vi "test_CCDSetRoi.vi"(0 "device selection":enum16{"monochromator", "CCD", "SCD"}(ring)=enum."CCD", 1 "Test should pass":bool=TRUE, 5 "set-up a connection":bool=TRUE, 9 "tear down connection":bool=TRUE, 11 "error in":errorcluster, 12 "activate logger?":bool, 13 "Handler Name":string="example logger handler") -> (2 "ready":bool, 3 "log-file path":path, 15 "error out":errorcluster)   [LabVIEW 2023]
uses:
  Classes/CCD/CCD.lvclass
  <vilib>/addons/_JKI Toolkits/Caraya/classes/Assert/Assert Not Error.vi
  <vilib>/addons/_JKI Toolkits/Caraya/classes/Test/Test.lvclass
  <vilib>/addons/_JKI Toolkits/Caraya/classes/Assert/Assert.lvclass
  C:/Projects/Horiba/horiba-labview-sdk/Source/Classes/GenericDevice/GenericDevice.lvclass
  C:/Projects/Horiba/horiba-labview-sdk/Source/Classes/CCD/CCD.lvclass
panel:
  in  "Delay between send and receive [ms]":i32=100
  out "config-JSON string":string
  # "Connector Pane"
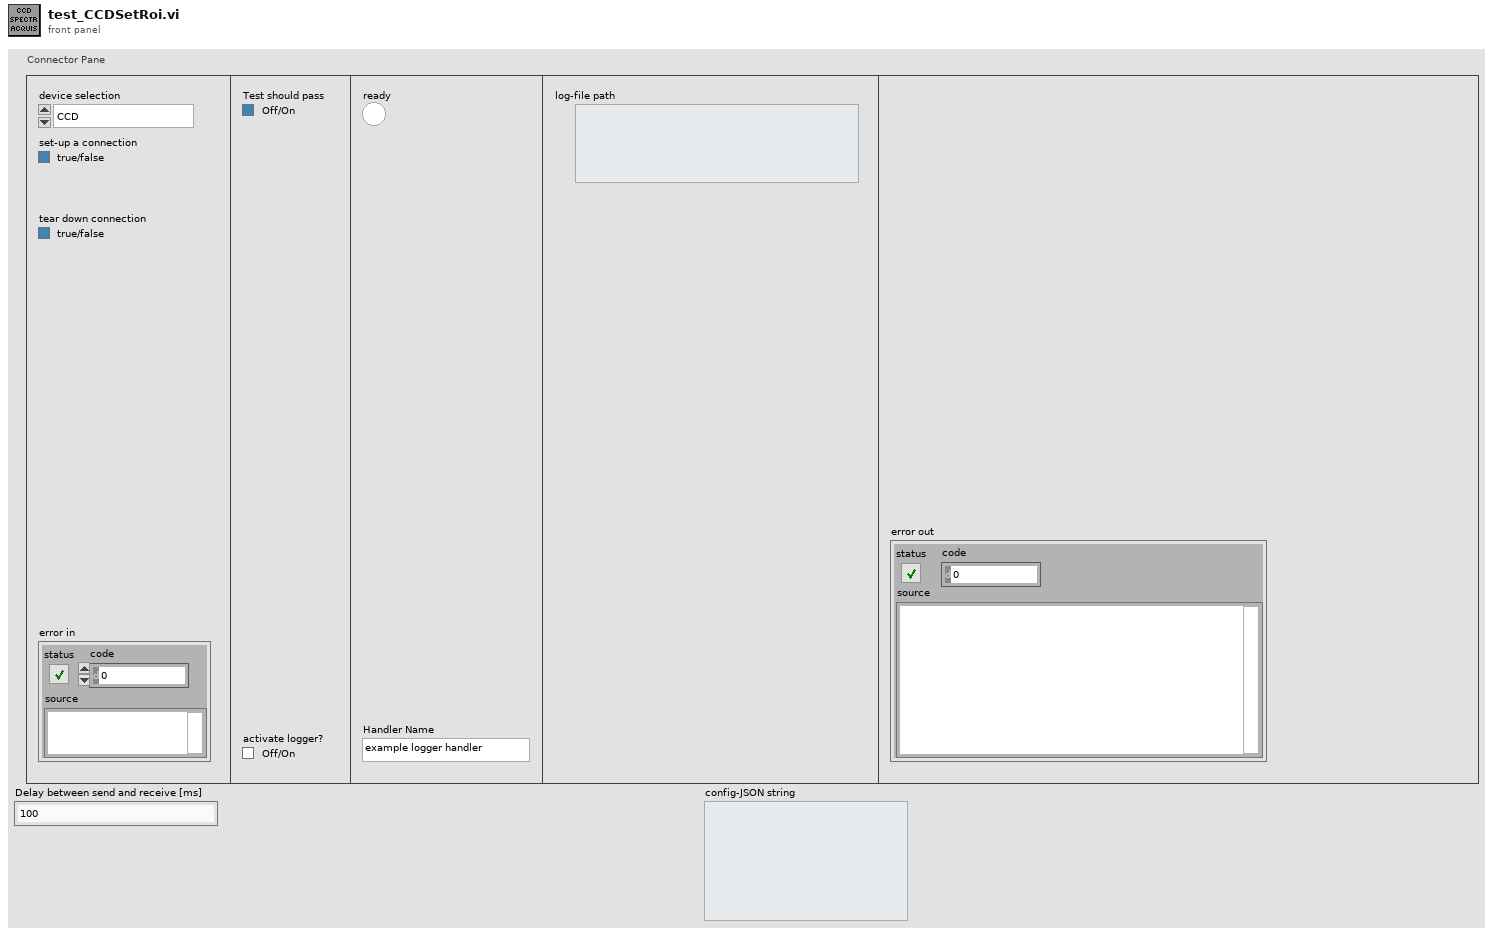
[diagram p1: front panel]
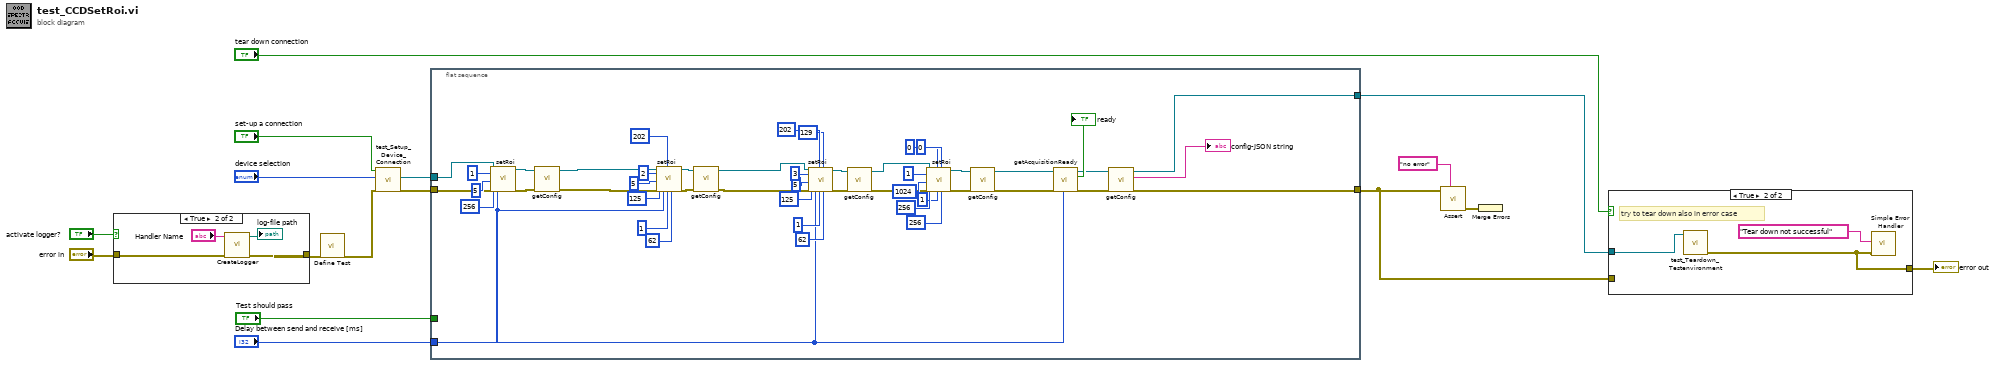
[diagram p0: block diagram]
diagram:
  n1 = case shown="True" "activate logger?" {
    tunnel: [w17 w20] -> w2
    tunnel: "error in" -> [w17 w21]
    frame False {
    }
    frame True {
      n2 = call "CreateLogger.vi"("error in (no error)"=w21, "Handler Name"="Handler Name") -> ("error out"=w20:errorcluster, "log-file path"=→"log-file path":path)  [unwired: 8 in]
    }
  }
  n3 = call <vilib>:"Define Test.vi"("error in (no error)"=w2) -> ("error out"=w7:errorcluster)  [unwired: 9 in, 1 out]
  n4 = call "test_Setup_Device_Connection.vi"("error in (no error)"=w7, "device selection"="device selection", "set-up a connection"="set-up a connection") -> ("error out"=w8:errorcluster, "CCD.lvclass"=w9:refnum<class "CCD.lvclass">)  [unwired: 5 in, 2 out]
  n5 = flat-sequence {
    tunnel: w8 -> [w52]
    tunnel: w9 -> [w36]
    tunnel: [w50] -> w12
    tunnel: "Test should pass" -> [w70]
    tunnel: [w48] -> w11
    tunnel: "Delay between send and receive [ms]" -> [w22]
    frame #0 {
      n6 = call "setRoi.vi"("CCD in"=w36, "ROI-index"=1, "xSize"=5, "ySize"=256, "error in (no error)"=w52, "Delay between send and receive [ms]"=w22) -> ("CCD out"=w40:refnum<class "CCD.lvclass">, "error out"=w39:errorcluster)  [unwired: 10 in, 2 out]
      n7 = call "getConfig.vi"("error in (no error)"=w39, "CCD in"=w40) -> ("error out"=w37:errorcluster, "CCD out"=w38:refnum<class "CCD.lvclass">)  [unwired: 7 in, 1 out]
      n8 = call "setRoi.vi"("CCD in"=w38, "ROI-index"=2, "xSize"=5, "ySize"=125, "error in (no error)"=w37, "Delay between send and receive [ms]"=w22, "xOrigin"=202, "xBin"=1, "yBin"=62) -> ("CCD out"=w43:refnum<class "CCD.lvclass">, "error out"=w44:errorcluster)  [unwired: 7 in, 2 out]
      n9 = call "getConfig.vi"("error in (no error)"=w44, "CCD in"=w43) -> ("error out"=w41:errorcluster, "CCD out"=w42:refnum<class "CCD.lvclass">)  [unwired: 7 in, 1 out]
      n10 = call "setRoi.vi"("CCD in"=w42, "ROI-index"=3, "xSize"=5, "ySize"=125, "error in (no error)"=w41, "Delay between send and receive [ms]"=w22, "xOrigin"=202, "xBin"=1, "yOrigin"=129, "yBin"=62) -> ("CCD out"=w45:refnum<class "CCD.lvclass">, "error out"=w46:errorcluster)  [unwired: 6 in, 2 out]
      n11 = call "getConfig.vi"("error in (no error)"=w46, "CCD in"=w45) -> ("error out"=w28:errorcluster, "CCD out"=w30:refnum<class "CCD.lvclass">)  [unwired: 7 in, 1 out]
      n12 = call "setRoi.vi"("CCD in"=w30, "ROI-index"=1, "xSize"=1024, "ySize"=256, "error in (no error)"=w28, "xOrigin"=0, "xBin"=1, "yOrigin"=0, "yBin"=256) -> ("CCD out"=w32:refnum<class "CCD.lvclass">, "error out"=w31:errorcluster)  [unwired: 7 in, 2 out]
      n13 = call "getConfig.vi"("error in (no error)"=w31, "CCD in"=w32) -> ("error out"=w27:errorcluster, "CCD out"=w29:refnum<class "CCD.lvclass">)  [unwired: 7 in, 1 out]
      n14 = call "getAcquisitionReady.vi"("Delay between send and receive [ms]"=w22, "error in (no error)"=w27, "CCD in"=w29) -> ("error out"=w51:errorcluster, "ready"=→"ready":bool, "CCD out"=w49:refnum<class "CCD.lvclass">)  [unwired: 6 in]
      n15 = call "getConfig.vi"("error in (no error)"=w51, "CCD in"=w49) -> ("error out"=w50:errorcluster, "config-JSON string"=→"config-JSON string":string, "CCD out"=w48:refnum<class "CCD.lvclass">)  [unwired: 7 in]
    }
  }
  n16 = call-poly <vilib>:"Assert.vi"("Label"="no error" ("Label (VI Title)"), "Not Error?"=w12) -> ("error out"=w14:errorcluster)  [unwired: 8 in, 1 out]
  n17 = Merge Errors(w14) -> ()  [unwired: 1 out]
  n18 = case shown="True" "tear down connection" {
    tunnel: w11 -> [_ w73]
    tunnel: [w71 w72] -> w10
    tunnel: w12 -> [w71 _]
    frame False {
    }
    frame True {
      # "try to tear down also in error case"
      n19 = call "test_Teardown_Testenvironment.vi"("GenericDevice.lvclass"=w73) -> ("error out"=w72:errorcluster)  [unwired: 9 in, 1 out]
      n20 = call <vilib>:"Simple Error Handler.vi"("error source (\" \")"="Tear down not successful" ("error source (\" \")"), "error in (no error)"=w72) -> ()  [unwired: 3 in, 5 out]
    }
  }
  "error out" <- w10
